vi "Get Optimiser Subpanel Values.vi"(0 "Optimiser SBlock in":refnum<class "Optimiser SBlock.lvclass">, 11 "error in (no error)":errorcluster) -> (4 "Optimiser SBlock out":refnum<class "Optimiser SBlock.lvclass">, 6 "Parameters - Numeric":T3[](array[typedef]), 8 "Parameters - String":T1[](array[typedef]), 10 "Observables":T2[](array[typedef]) {"Weight" min=0.0 max=1.0}, 14 "Number of Exploration Runs":i32, 15 "error out":errorcluster)   [LabVIEW 2020, in "CIRCUS_uServices.lvlib" / "Run Utilities.lvlib" / "Optimiser SBlock.lvclass"]
uses:
  Optimiser SBlock.lvclass
  Optimiser SBlock.lvclass/Optimiser SBlock.ctl
  Optimiser Cell/Optimise parameter - numeric.ctl
  Optimiser Cell/Optimiser Cell.lvclass
  Optimiser Cell/Optimisation observable.ctl
  Optimiser Cell/Optimise parameter - string.ctl
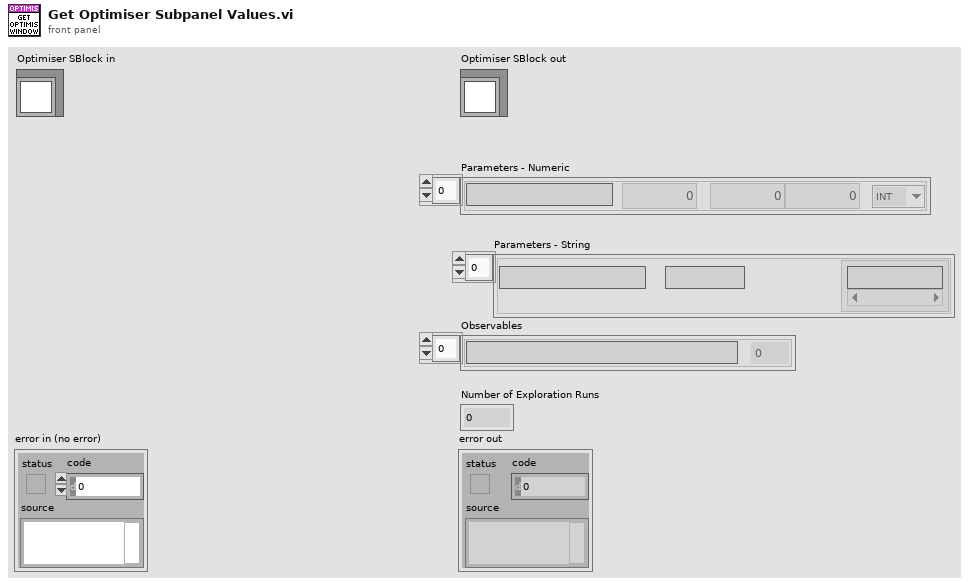
[diagram p1: front panel]
types:
  T1 = typedef "CIRCUS_uServices.lvlib/Run Utilities.lvlib/Optimiser Cell.lvclass/Optimise parameter - string.ctl" = cluster{"Name":string, "Start value":string, "Options":string[]}
  T2 = typedef "CIRCUS_uServices.lvlib/Run Utilities.lvlib/Optimiser Cell.lvclass/Optimisation observable.ctl" = cluster{"Name":string, "Weight":dbl}
  T3 = typedef "CIRCUS_uServices.lvlib/Run Utilities.lvlib/Optimiser Cell.lvclass/Optimise parameter - numeric.ctl" = cluster{"Name":string, "Start value":dbl, "From":dbl, "To":dbl, "dtype":enum16{"INT", "DBL"}}
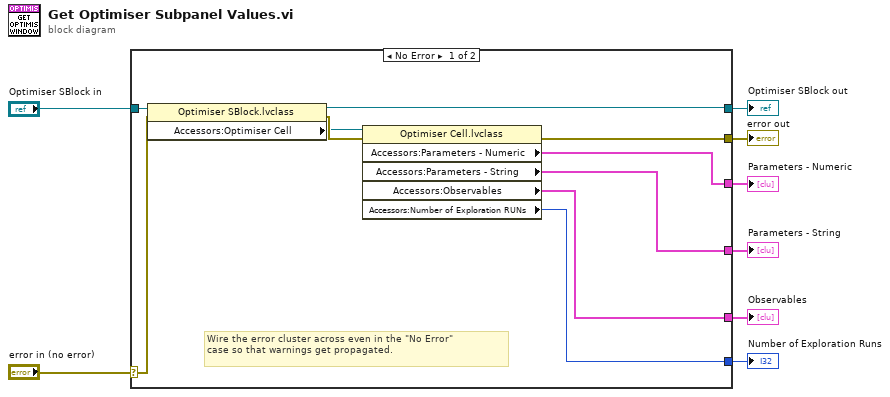
[diagram p0: block diagram]
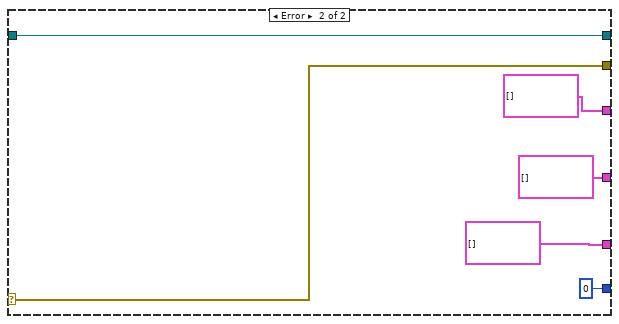
[diagram p2: hidden frame]
diagram:
  n1 = case shown="No Error" "error in (no error)" {
    selector: "error in (no error)" -> [w14 w24]
    tunnel: [w10 w24] -> w7
    tunnel: [w16 w23] -> w6
    tunnel: "Optimiser SBlock in" -> [w17 w23]
    tunnel: [w13 T3[] [] ("Parameters")] -> w4
    tunnel: [w12 T2[] [] ("Observables")] -> w3
    tunnel: [w11 0 ("Number of Exploration Runs")] -> w2
    tunnel: [w9 T1[] [] ("Accessors:Optimiser.Parameters - String")] -> w1
    frame No Error {
      # "Wire the error cluster across even in the \"No Error\"\ncase so that warnings get propagated."
      n2 = property class="Optimiser SBlock.lvclass"(reference=w17, error in=w14) -> (reference out=w16:refnum<class "Optimiser SBlock.lvclass">, error out=w18:errorcluster, "Accessors:Optimiser Cell"=w15:refnum<class "Optimiser Cell.lvclass">)
      n3 = property class="Optimiser Cell.lvclass"(reference=w15, error in=w18) -> (error out=w10:errorcluster, "Accessors:Parameters - Numeric"=w13:T3[], "Accessors:Parameters - String"=w9:T1[], "Accessors:Observables"=w12:T2[], "Accessors:Number of Exploration RUNs"=w11:i32)  [unwired: 1 out]
    }
    frame Error {
    }
  }
  "error out" <- w7
  "Optimiser SBlock out" <- w6
  "Parameters - Numeric" <- w4
  "Observables" <- w3
  "Number of Exploration Runs" <- w2
  "Parameters - String" <- w1
